vi "logicTest.vi"() -> ()   [LabVIEW 2022 SP3]
panel:
  in  "stop":bool
  in  "Port 2":string="60"
  in  "two notes":bool
  in  "note (input a number) 2":string="60"
  in  "sensor 2":u16(ring)=1 items=["", "Touch Sensor", "Color Sensor"]
  out "concatenated string":string
  in  "Port":string="60"
  in  "note (input a number)":string="60"
  in  "sensor":u16(ring)=1 items=["Touch Sensor"=1, "Color Sensor"=2]
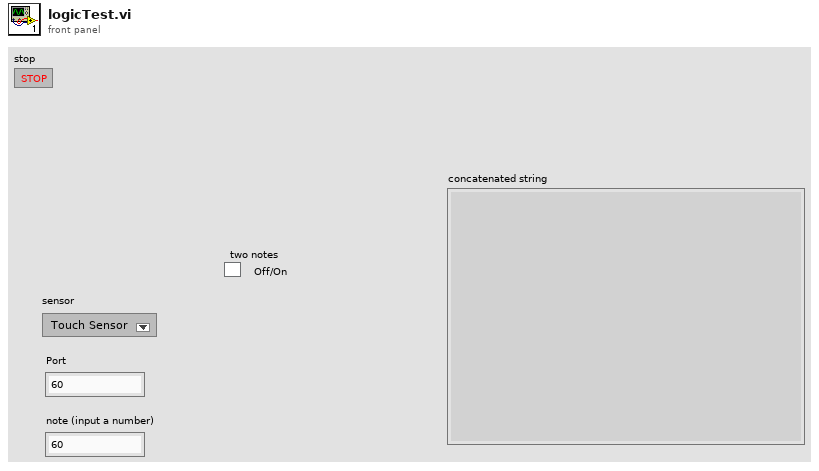
[diagram p1: front panel]
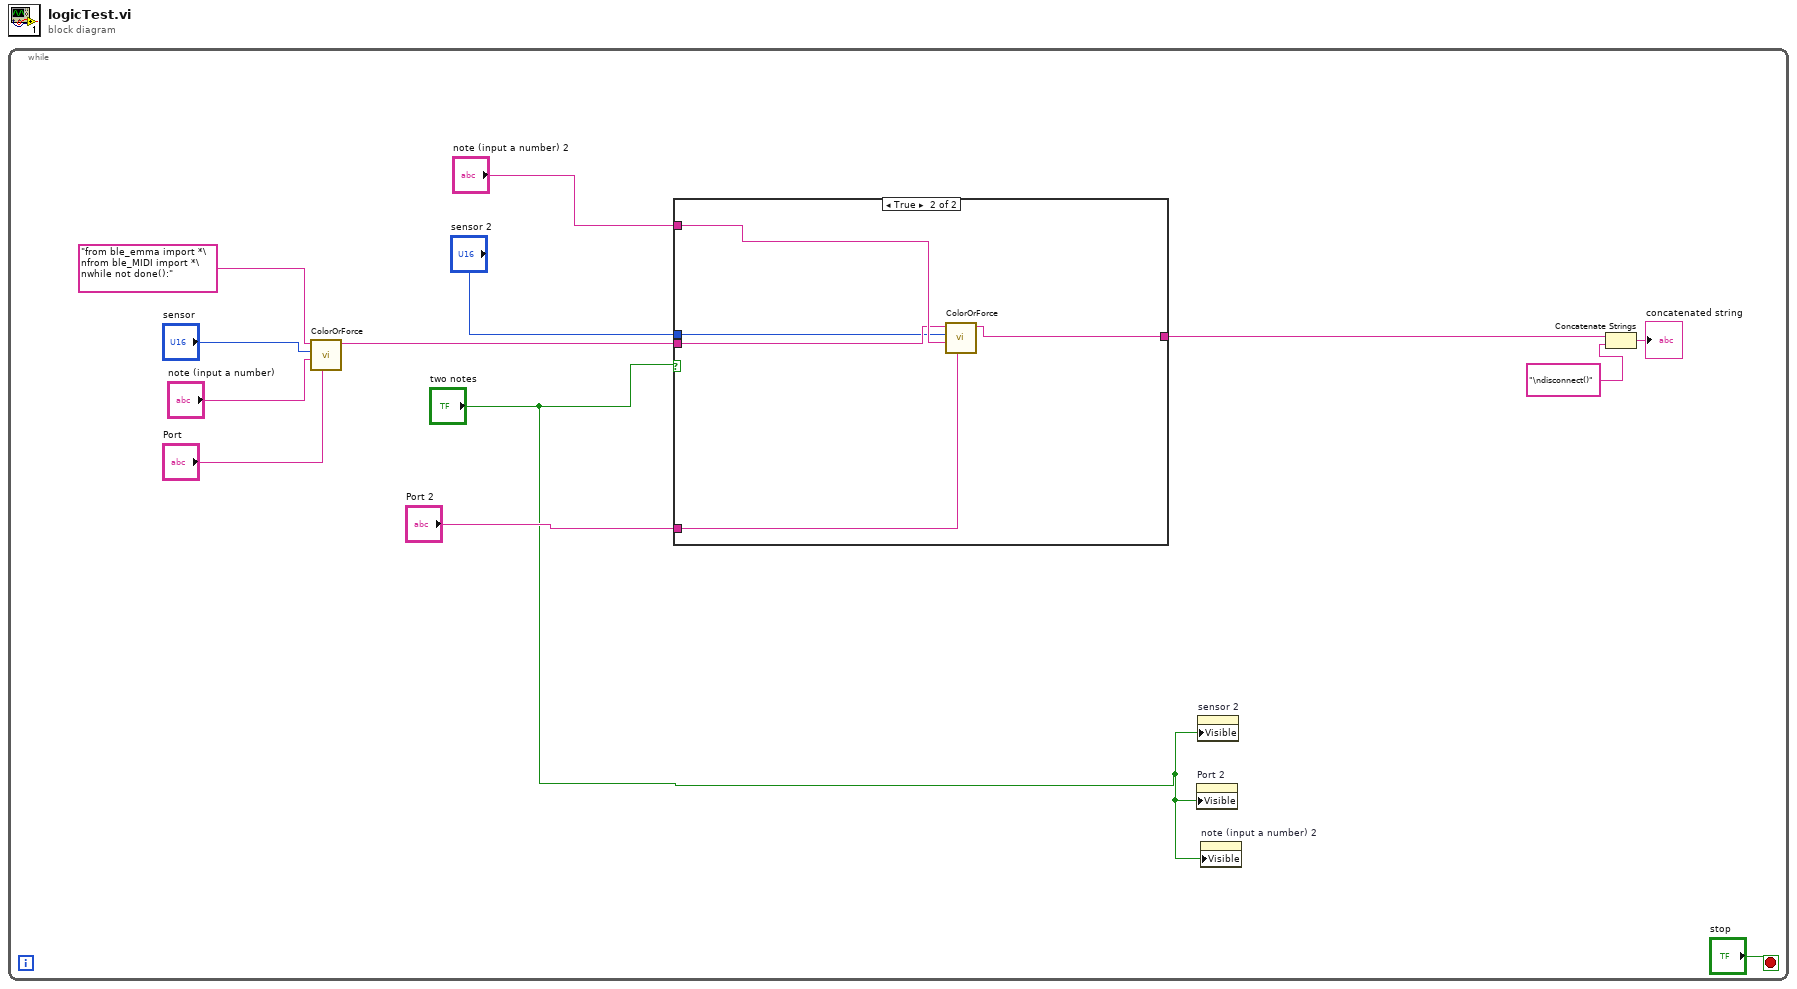
[diagram p0: block diagram]
diagram:
  n1 = while {
    stop <- "stop" stop-if-true
    n2 = call "ColorOrForce.vi"("Port"="Port", "note (input a number)"="note (input a number)", "sensor"="sensor", "String in"="from ble_emma import *\nfrom ble_MIDI import *\nwhile not done():") -> ("String out"=w7:string)  [unwired: 7 in]
    n3 = case shown="True" "two notes" {
      tunnel: w7 -> [w14 w18]
      tunnel: [w14 w15] -> w6
      tunnel: "note (input a number) 2" -> [_ w19]
      tunnel: "Port 2" -> [_ w17]
      tunnel: "sensor 2" -> [_ w16]
      frame False {
      }
      frame True {
        n4 = call "ColorOrForce.vi"("Port"=w17, "note (input a number)"=w19, "sensor"=w16, "String in"=w18) -> ("String out"=w15:string)  [unwired: 7 in]
      }
    }
    n5 = property on="Port 2" class="Str"("Visible"="two notes") -> ()  [unwired: 2 in, 2 out]
    n6 = property on="sensor 2" class="Ring (strict)"("Visible"="two notes") -> ()  [unwired: 2 in, 2 out]
    n7 = property on="note (input a number) 2" class="Str"("Visible"="two notes") -> ()  [unwired: 2 in, 2 out]
    n8 = Concatenate Strings(w6, "\ndisconnect()" ("string")) -> (→"concatenated string":string)
  }
